vi "Read lifter config_Running info.vi"(4 "error in (no error)":errorcluster) -> (0 "error out":errorcluster, 3 "Current insert name":string)   [LabVIEW 2019]
uses:
  <vilib>/Utility/config.llb/Read Key (String).vi
  <vilib>/Utility/config.llb/NI_LVConfig.lvlib
panel:
  out "appended path":path
  out "concatenated string":string
  in  "File Name":string="Lifter config"
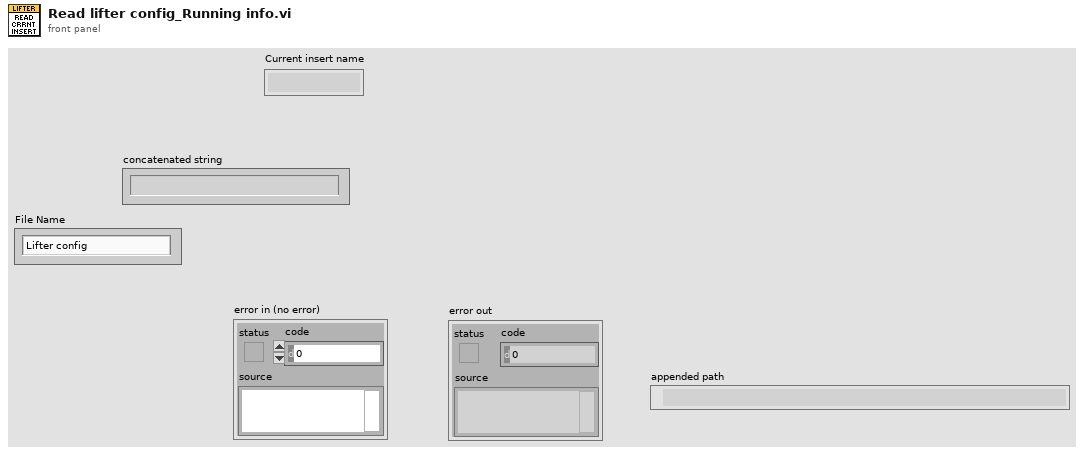
[diagram p1: front panel]
types:
  T1 = typedef "NI_LVConfig.lvlib/Config Data RefNum.ctl" = refnum<k1>
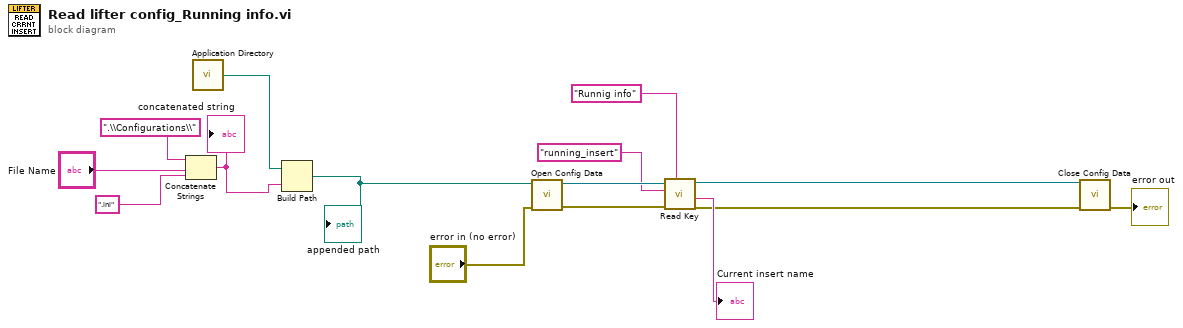
[diagram p0: block diagram]
diagram:
  n1 = Concatenate Strings(".\\Configurations\\" ("string"), "File Name", ".ini" ("string")) -> (w13:string)
  "concatenated string" <- w13
  n2 = call <vilib>:"Application Directory.vi"() -> ("Application Directory"=w11:path)
  n3 = Build Path(base path=w11, name or relative path=w13) -> (appended path=w8:path)
  "appended path" <- w8
  n4 = call <vilib>:"Open Config Data.vi"("error in (no error)"="error in (no error)", "configuration file path"=w8) -> ("error out"=w6:errorcluster, "refnum"=w7:T1)  [unwired: 7 in, 1 out]
  n5 = call-poly <vilib>:"Read Key.vi"("section"="Runnig info", "error in (no error)"=w6, "key"="running_insert" ("section"), "refnum"=w7) -> ("error out"=w2:errorcluster, "value"=→"Current insert name":string, "refnum out"=w1:T1)  [unwired: 4 in, 1 out]
  n6 = call <vilib>:"Close Config Data.vi"("error in (no error)"=w2, "refnum"=w1) -> ("error out"=→"error out":errorcluster)  [unwired: 8 in, 1 out]
